vi "CRYTS Step Remove.vi"(9 "Harware or Calibration":bool, 11 "Tree Sequence":refnum<vi>) -> (2 "bResult":bool, 3 "Tree Sequence Ref Out":refnum<vi>)   [LabVIEW 2013]
uses:
  CRYStepSetup/CRYStepSetup Global.vi
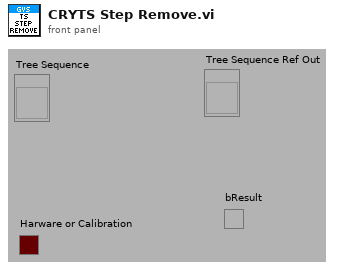
[diagram p1: front panel]
types:
  T1 = enum16{"Insert", "Remove", "Move up", "Move down"}
  T2 = cluster{"SourceRowNum":i32, "SourceCount":i32, "TargetRowNum":i32, "bResult":bool, "EditRowNum":i32}
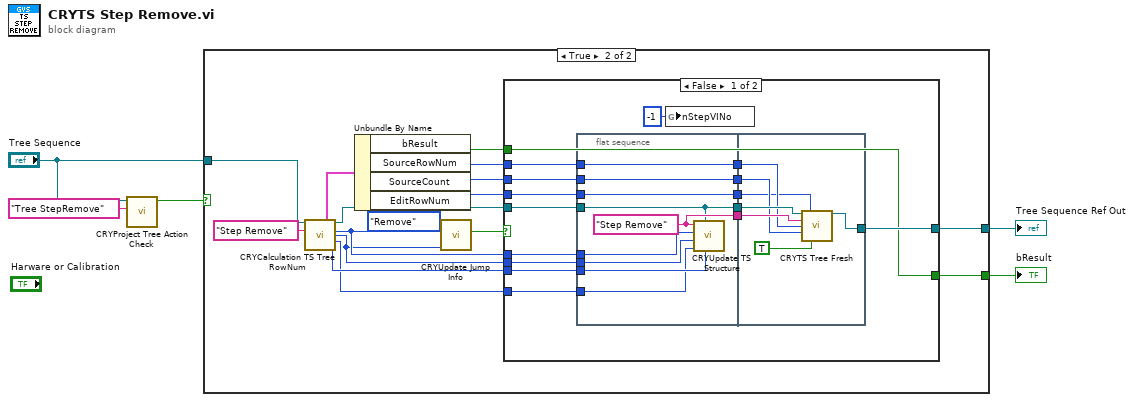
[diagram p0: block diagram]
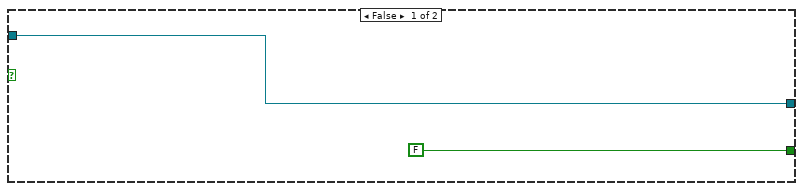
[diagram p2: hidden frame]
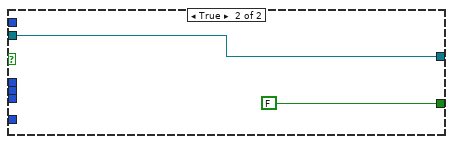
[diagram p3: hidden frame]
diagram:
  n1 = call "CRYProject Tree Action Check.vi"("sOption"="Tree StepRemove", "Project Tree reference"="Tree Sequence") -> ("bResult"=w4:bool)  [unwired: 8 in, 1 out]
  n2 = case shown="True" w4 {
    tunnel: "Tree Sequence" -> [w6 w23]
    tunnel: [FALSE ("Boolean") w13] -> w3
    tunnel: [w6 w16] -> w1
    frame False {
    }
    frame True {
      n3 = call "CRYCalculation TS Tree RowNum.vi"("Tree Task SequenceIn"=w23, "sOption"="Step Remove") -> ("DispInfo Cluster Out"=w12:T2, "Tree Task Sequence Out"=w17:refnum<vi>, "SourceRowNum"=w22:i32, "SourceCount"=w21:i32, "TargetRowNum"=w14:i32, "EditRowNum"=w20:i32)  [unwired: 7 in, 1 out]
      n4 = Unbundle By Name(w12) -> ("bResult"=w11:bool, "SourceRowNum"=w10:i32, "SourceCount"=w9:i32, "EditRowNum"=w8:i32)
      n5 = call "CRYUpdate Jump Info.vi"("SourceCount"=w21, "Step number Selected"=w22, "Action"=T1."Remove") -> ("Canceled?"=w15:bool)  [unwired: 7 in, 1 out]
      n6 = case shown="False" w15 {
        tunnel: w22 -> [w38 _]
        tunnel: w21 -> [w37 _]
        tunnel: w20 -> [w36 _]
        tunnel: w17 -> [w35 w57]
        tunnel: [w34 w57] -> w16
        tunnel: [w31 FALSE ("Boolean")] -> w13
        tunnel: w14 -> [w32 _]
        tunnel: w11 -> [w31 _]
        tunnel: w10 -> [w29 _]
        tunnel: w9 -> [w27 _]
        tunnel: w8 -> [w25 _]
        frame False {
          n7 = flat-sequence {
            tunnel: w38 -> [w46]
            tunnel: w37 -> [w45]
            tunnel: w36 -> [w48]
            tunnel: w35 -> [w40]
            tunnel: [w40] -> w39
            tunnel: [w47] -> w33
            tunnel: w32 -> [w44]
            tunnel: [w43] -> w30
            tunnel: w29 -> [w43]
            tunnel: [w42] -> w28
            tunnel: w27 -> [w42]
            tunnel: [w41] -> w26
            tunnel: w25 -> [w41]
            tunnel: w39 -> [w54]
            tunnel: [w53] -> w34
            tunnel: w33 -> [w52]
            tunnel: w30 -> [w51]
            tunnel: w28 -> [w50]
            tunnel: w26 -> [w49]
            frame #0 {
              w47 = "Step Remove" ("sOption")
              n8 = call "CRYUpdate TS Structure.vi"("Edit Step Num"=w48, "Tree Task SequenceIn"=w40, "Target Index"=w44, "Count"=w45, "Source Index"=w46, "sOption"=w47) -> ()  [unwired: 6 in]
            }
            frame #1 {
              n9 = call "CRYTS Tree Fresh.vi"("SequenceTree"=w54, "Edit Index"=w49, "sOption"=w52, "Source Index"=w51, "SourceCount"=w50, "Is Refresh?"=TRUE) -> ("SequenceTree out"=w53:refnum<vi>)  [unwired: 9 in]
            }
          }
          n10 = global write "CRYStepSetup Global.vi" "nStepVINo"(-1 ("nStepVINo")) -> ()
        }
        frame True {
        }
      }
    }
  }
  "Tree Sequence Ref Out" <- w1
  "bResult" <- w3
